vi "Compile Settings.vi"(8 "error in":errorcluster, 10 "Settings(JSON)":string, 11 "iPluginSettings in":refnum<class "Template Deployment Hooks.lvclass">) -> (0 "error out":errorcluster, 2 "Compiled Settings":variant, 3 "iPluginSettings out":refnum<class "Template Deployment Hooks.lvclass">)   [LabVIEW 2026, in "Template Deployment Hooks.lvlib" / "Template Deployment Hooks.lvclass"]
uses:
  Template Deployment Hooks.lvclass
  Template Deployment Hooks.lvclass/Template Deployment Hooks.ctl
  <vilib>/JDP Science/JSONtext/JSONtext.lvlib
  Shared/Compiled.Settings.ctl
  Shared/GroupedChannel.ctl
  Shared/GroupedChannelRefs.ctl
  Template Deployment Hooks.lvlib
  Shared/PluginSettings.ctl
  Shared/GroupSettings.ctl
  Shared/ChannelGroups.ctl
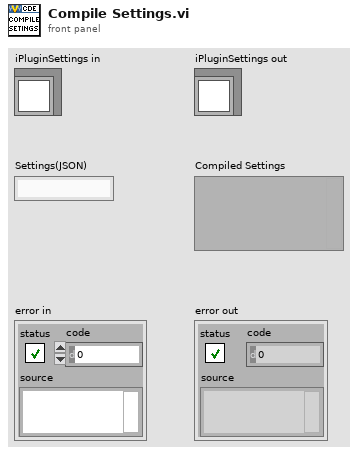
[diagram p1: front panel]
types:
  T1 = typedef "Compiled.Settings.ctl" = cluster{"Plugin Settings":T2, "Channel Groups":T3}
  T2 = typedef "PluginSettings.ctl" = cluster{"ExampleCustomDevice":cluster{"Name":string, "Properties":cluster{"Low frequency":string, "Low frequency (Hz)":bool[], "High frequency [Hz]":bool, "Frequency : Low Level frequency":dbl[], "Frequency.High frequency":dbl, "I16_PropertyExample":i16, "I16ArrayPropertyExample":i16[], "I32PropertyExample":i32, "I32ArrayPropertyExample":i32[], "I64PropertyExample":i64, "I64ArrayPropertyExample":i64[], "StringArrayPropertyExample":string[], "StringPropertyExample":string, "U16PropertyExample":u16, "U16ArrayPropertyExample":u16[], "U32PropertyExample":u32, "U32ArrayPropertyExample":u32[], "U64PropertyExample":u64, "U64ArrayPropertyExample":u64[], "DependentFilePropertyExample":cluster{"Version":string, "Type":string, "ForceDownload":bool, "RTDestination":string, "SupportedTarget":string, "MD5":string, "Path":string}, "VariantPropertyExample":variant, "TargetOS":string, "TargetRate":dbl}, "Channels":cluster{"TimeChannel":cluster{"Name":string, "Properties":cluster{"Low frequency":string, "Low frequency (Hz)":bool[], "High frequency [Hz]":bool, "Frequency : Low Level frequency":dbl[], "Frequency.High frequency":dbl, "I16PropertyExample":i16, "I16ArrayPropertyExample":i16[], "I32PropertyExample":i32, "I32ArrayPropertyExample":i32[], "I64PropertyExample":i64, "I64ArrayPropertyExample":i64[], "StringArrayPropertyExample":string[], "StringPropertyExample":string, "U16PropertyExample":u16, "U16ArrayPropertyExample":u16[], "U32PropertyExample":u32, "U32ArrayPropertyExample":u32[], "U64PropertyExample":u64, "U64ArrayPropertyExample":u64[], "DependentFilePropertyExample":cluster{"Version":string, "Type":string, "ForceDownload":bool, "RTDestination":string, "SupportedTarget":string, "MD5":string, "Path":string}, "VariantPropertyExample":variant}, "DefaultValue":dbl, "Units":string, "GroupName":string, "Type":string, "Faultable":bool, "Scalable":bool, "ChannelDataReference":i32}[], "FrequencyChannel":cluster{"Name":string, "Properties":cluster{"BinaryStringPropertyExample":string, "BooleanArrayPropertyExample":bool[], "BooleanPropertyExample":bool, "DoubleArrayPropertyExample":dbl[], "DoublePropertyExample":dbl, "I16PropertyExample":i16, "I16ArrayPropertyExample":i16[], "I32PropertyExample":i32, "I32ArrayPropertyExample":i32[], "I64PropertyExample":i64, "I64ArrayPropertyExample":i64[], "StringArrayPropertyExample":string[], "StringPropertyExample":string, "U16PropertyExample":u16, "U16ArrayPropertyExample":u16[], "U32PropertyExample":u32, "U32ArrayPropertyExample":u32[], "U64PropertyExample":u64, "U64ArrayPropertyExample":u64[], "DependentFilePropertyExample":cluster{"Version":string, "Type":string, "ForceDownload":bool, "RTDestination":string, "SupportedTarget":string, "MD5":string, "Path":string}, "VariantPropertyExample":variant}, "DefaultValue":dbl, "Units":string, "GroupName":string, "Type":string, "Faultable":bool, "Scalable":bool, "ChannelDataReference":i32}[]}, "Waveforms":cluster{"AnalogInput":cluster{"Name":string, "Properties":cluster{"Low frequency":string, "Low frequency (Hz)":bool[], "High frequency [Hz]":bool, "Frequency : Low Level frequency":dbl[], "Frequency.High frequency":dbl, "I16PropertyExample":i16, "I16ArrayPropertyExample":i16[], "I32PropertyExample":i32, "I32ArrayPropertyExample":i32[], "I64PropertyExample":i64, "I64ArrayPropertyExample":i64[], "StringArrayPropertyExample":string[], "StringPropertyExample":string, "U16PropertyExample":u16, "U16ArrayPropertyExample":u16[], "U32PropertyExample":u32, "U32ArrayPropertyExample":u32[], "U64PropertyExample":u64, "U64ArrayPropertyExample":u64[], "DependentFilePropertyExample":cluster{"Version":string, "Type":string, "ForceDownload":bool, "RTDestination":string, "SupportedTarget":string, "MD5":string, "Path":string}, "VariantPropertyExample":variant}, "DataType":string, "Units":string, "WaveformDataReference":i32}[]}, "Sections":cluster{"SectionA0":cluster{"Name":string, "Properties":cluster{"BinaryStringPropertyExample":string, "BooleanArrayPropertyExample":bool[], "BooleanPropertyExample":bool, "DoubleArrayPropertyExample":dbl[], "DoublePropertyExample":dbl, "I16PropertyExample":i16, "I16ArrayPropertyExample":i16[], "I32PropertyExample":i32, "I32ArrayPropertyExample":i32[], "I64PropertyExample":i64, "I64ArrayPropertyExample":i64[], "StringArrayPropertyExample":string[], "StringPropertyExample":string, "U16PropertyExample":u16, "U16ArrayPropertyExample":u16[], "U32PropertyExample":u32, "U32ArrayPropertyExample":u32[], "U64PropertyExample":u64, "U64ArrayPropertyExample":u64[], "DependentFilePropertyExample":cluster{"Version":string, "Type":string, "ForceDownload":bool, "RTDestination":string, "SupportedTarget":string, "MD5":string, "Path":string}, "VariantPropertyExample":variant}, "Channels":cluster{"TimeChannel":cluster{"Name":string, "Properties":cluster{"Low frequency":string, "Low frequency (Hz)":bool[], "High frequency [Hz]":bool, "Frequency : Low Level frequency":dbl[], "Frequency.High frequency":dbl, "I16PropertyExample":i16, "I16ArrayPropertyExample":i16[], "I32PropertyExample":i32, "I32ArrayPropertyExample":i32[], "I64PropertyExample":i64, "I64ArrayPropertyExample":i64[], "StringArrayPropertyExample":string[], "StringPropertyExample":string, "U16PropertyExample":u16, "U16ArrayPropertyExample":u16[], "U32PropertyExample":u32, "U32ArrayPropertyExample":u32[], "U64PropertyExample":u64, "U64ArrayPropertyExample":u64[], "DependentFilePropertyExample":cluster{"Version":string, "Type":string, "ForceDownload":bool, "RTDestination":string, "SupportedTarget":string, "MD5":string, "Path":string}, "VariantPropertyExample":variant}, "DefaultValue":dbl, "Units":string, "GroupName":string, "Type":string, "Faultable":bool, "Scalable":bool, "ChannelDataReference":i32}[], "FrequencyChannel":cluster{"Name":string, "Properties":cluster{"BinaryStringPropertyExample":string, "BooleanArrayPropertyExample":bool[], "BooleanPropertyExample":bool, "DoubleArrayPropertyExample":dbl[], "DoublePropertyExample":dbl, "I16PropertyExample":i16, "I16ArrayPropertyExample":i16[], "I32PropertyExample":i32, "I32ArrayPropertyExample":i32[], "I64PropertyExample":i64, "I64ArrayPropertyExample":i64[], "StringArrayPropertyExample":string[], "StringPropertyExample":string, "U16PropertyExample":u16, "U16ArrayPropertyExample":u16[], "U32PropertyExample":u32, "U32ArrayPropertyExample":u32[], "U64PropertyExample":u64, "U64ArrayPropertyExample":u64[], "DependentFilePropertyExample":cluster{"Version":string, "Type":string, "ForceDownload":bool, "RTDestination":string, "SupportedTarget":string, "MD5":string, "Path":string}, "VariantPropertyExample":variant}, "DefaultValue":dbl, "Units":string, "GroupName":string, "Type":string, "Faultable":bool, "Scalable":bool, "ChannelDataReference":i32}[]}, "Waveforms":cluster{"AnalogInput":cluster{"Name":string, "Properties":cluster{"Low frequency":string, "Low frequency (Hz)":bool[], "High frequency [Hz]":bool, "Frequency : Low Level frequency":dbl[], "Frequency.High frequency":dbl, "I16PropertyExample":i16, "I16ArrayPropertyExample":i16[], "I32PropertyExample":i32, "I32ArrayPropertyExample":i32[], "I64PropertyExample":i64, "I64ArrayPropertyExample":i64[], "StringArrayPropertyExample":string[], "StringPropertyExample":string, "U16PropertyExample":u16, "U16ArrayPropertyExample":u16[], "U32PropertyExample":u32, "U32ArrayPropertyExample":u32[], "U64PropertyExample":u64, "U64ArrayPropertyExample":u64[], "DependentFilePropertyExample":cluster{"Version":string, "Type":string, "ForceDownload":bool, "RTDestination":string, "SupportedTarget":string, "MD5":string, "Path":string}, "VariantPropertyExample":variant}, "DataType":string, "Units":string, "WaveformDataReference":i32}[]}}[], "SectionR1":cluster{"Name":string, "Properties":cluster{"Low frequency":string, "Low frequency (Hz)":bool[], "High frequency [Hz]":bool, "Frequency : Low Level frequency":dbl[], "Frequency.High frequency":dbl, "I16PropertyExample":i16, "I16ArrayPropertyExample":i16[], "I32PropertyExample":i32, "I32ArrayPropertyExample":i32[], "I64PropertyExample":i64, "I64ArrayPropertyExample":i64[], "StringArrayPropertyExample":string[], "StringPropertyExample":string, "U16PropertyExample":u16, "U16ArrayPropertyExample":u16[], "U32PropertyExample":u32, "U32ArrayPropertyExample":u32[], "U64PropertyExample":u64, "U64ArrayPropertyExample":u64[], "DependentFilePropertyExample":cluster{"Version":string, "Type":string, "ForceDownload":bool, "RTDestination":string, "SupportedTarget":string, "MD5":string, "Path":string}, "VariantPropertyExample":variant}, "Channels":cluster{"TimeChannel":cluster{"Name":string, "Properties":cluster{"Low frequency":string, "Low frequency (Hz)":bool[], "High frequency [Hz]":bool, "Frequency : Low Level frequency":dbl[], "Frequency.High frequency":dbl, "I16PropertyExample":i16, "I16ArrayPropertyExample":i16[], "I32PropertyExample":i32, "I32ArrayPropertyExample":i32[], "I64PropertyExample":i64, "I64ArrayPropertyExample":i64[], "StringArrayPropertyExample":string[], "StringPropertyExample":string, "U16PropertyExample":u16, "U16ArrayPropertyExample":u16[], "U32PropertyExample":u32, "U32ArrayPropertyExample":u32[], "U64PropertyExample":u64, "U64ArrayPropertyExample":u64[], "DependentFilePropertyExample":cluster{"Version":string, "Type":string, "ForceDownload":bool, "RTDestination":string, "SupportedTarget":string, "MD5":string, "Path":string}, "VariantPropertyExample":variant}, "DefaultValue":dbl, "Units":string, "GroupName":string, "Type":string, "Faultable":bool, "Scalable":bool, "ChannelDataReference":i32}[], "FrequencyChannel":cluster{"Name":string, "Properties":cluster{"BinaryStringPropertyExample":string, "BooleanArrayPropertyExample":bool[], "BooleanPropertyExample":bool, "DoubleArrayPropertyExample":dbl[], "DoublePropertyExample":dbl, "I16PropertyExample":i16, "I16ArrayPropertyExample":i16[], "I32PropertyExample":i32, "I32ArrayPropertyExample":i32[], "I64PropertyExample":i64, "I64ArrayPropertyExample":i64[], "StringArrayPropertyExample":string[], "StringPropertyExample":string, "U16PropertyExample":u16, "U16ArrayPropertyExample":u16[], "U32PropertyExample":u32, "U32ArrayPropertyExample":u32[], "U64PropertyExample":u64, "U64ArrayPropertyExample":u64[], "DependentFilePropertyExample":cluster{"Version":string, "Type":string, "ForceDownload":bool, "RTDestination":string, "SupportedTarget":string, "MD5":string, "Path":string}, "VariantPropertyExample":variant}, "DefaultValue":dbl, "Units":string, "GroupName":string, "Type":string, "Faultable":bool, "Scalable":bool, "ChannelDataReference":i32}[]}, "Sections":cluster{"SectionA0":cluster{"Name":string, "Properties":cluster{"BinaryStringPropertyExample":string, "BooleanArrayPropertyExample":bool[], "BooleanPropertyExample":bool, "DoubleArrayPropertyExample":dbl[], "DoublePropertyExample":dbl, "I16PropertyExample":i16, "I16ArrayPropertyExample":i16[], "I32PropertyExample":i32, "I32ArrayPropertyExample":i32[], "I64PropertyExample":i64, "I64ArrayPropertyExample":i64[], "StringArrayPropertyExample":string[], "StringPropertyExample":string, "U16PropertyExample":u16, "U16ArrayPropertyExample":u16[], "U32PropertyExample":u32, "U32ArrayPropertyExample":u32[], "U64PropertyExample":u64, "U64ArrayPropertyExample":u64[], "DependentFilePropertyExample":cluster{"Version":string, "Type":string, "ForceDownload":bool, "RTDestination":string, "SupportedTarget":string, "MD5":string, "Path":string}, "VariantPropertyExample":variant}, "Channels":cluster{"TimeChannel":cluster{"Name":string, "Properties":cluster{"Low frequency":string, "Low frequency (Hz)":bool[], "High frequency [Hz]":bool, "Frequency : Low Level frequency":dbl[], "Frequency.High frequency":dbl, "I16PropertyExample":i16, "I16ArrayPropertyExample":i16[], "I32PropertyExample":i32, "I32ArrayPropertyExample":i32[], "I64PropertyExample":i64, "I64ArrayPropertyExample":i64[], "StringArrayPropertyExample":string[], "StringPropertyExample":string, "U16PropertyExample":u16, "U16ArrayPropertyExample":u16[], "U32PropertyExample":u32, "U32ArrayPropertyExample":u32[], "U64PropertyExample":u64, "U64ArrayPropertyExample":u64[], "DependentFilePropertyExample":cluster{"Version":string, "Type":string, "ForceDownload":bool, "RTDestination":string, "SupportedTarget":string, "MD5":string, "Path":string}, "VariantPropertyExample":variant}, "DefaultValue":dbl, "Units":string, "GroupName":string, "Type":string, "Faultable":bool, "Scalable":bool, "ChannelDataReference":i32}[], "FrequencyChannel":cluster{"Name":string, "Properties":cluster{"BinaryStringPropertyExample":string, "BooleanArrayPropertyExample":bool[], "BooleanPropertyExample":bool, "DoubleArrayPropertyExample":dbl[], "DoublePropertyExample":dbl, "I16PropertyExample":i16, "I16ArrayPropertyExample":i16[], "I32PropertyExample":i32, "I32ArrayPropertyExample":i32[], "I64PropertyExample":i64, "I64ArrayPropertyExample":i64[], "StringArrayPropertyExample":string[], "StringPropertyExample":string, "U16PropertyExample":u16, "U16ArrayPropertyExample":u16[], "U32PropertyExample":u32, "U32ArrayPropertyExample":u32[], "U64PropertyExample":u64, "U64ArrayPropertyExample":u64[], "DependentFilePropertyExample":cluster{"Version":string, "Type":string, "ForceDownload":bool, "RTDestination":string, "SupportedTarget":string, "MD5":string, "Path":string}, "VariantPropertyExample":variant}, "DefaultValue":dbl, "Units":string, "GroupName":string, "Type":string, "Faultable":bool, "Scalable":bool, "ChannelDataReference":i32}[]}, "Waveforms":cluster{"AnalogInput":cluster{"Name":string, "Properties":cluster{"Low frequency":string, "Low frequency (Hz)":bool[], "High frequency [Hz]":bool, "Frequency : Low Level frequency":dbl[], "Frequency.High frequency":dbl, "I16PropertyExample":i16, "I16ArrayPropertyExample":i16[], "I32PropertyExample":i32, "I32ArrayPropertyExample":i32[], "I64PropertyExample":i64, "I64ArrayPropertyExample":i64[], "StringArrayPropertyExample":string[], "StringPropertyExample":string, "U16PropertyExample":u16, "U16ArrayPropertyExample":u16[], "U32PropertyExample":u32, "U32ArrayPropertyExample":u32[], "U64PropertyExample":u64, "U64ArrayPropertyExample":u64[], "DependentFilePropertyExample":cluster{"Version":string, "Type":string, "ForceDownload":bool, "RTDestination":string, "SupportedTarget":string, "MD5":string, "Path":string}, "VariantPropertyExample":variant}, "DataType":string, "Units":string, "WaveformDataReference":i32}[]}}[]}}[]}}}
  T3 = typedef "ChannelGroups.ctl" = cluster{"Channel Refs":T4, "Group Settings":T5[]}
  T4 = typedef "GroupedChannelRefs.ctl" = cluster{"Read":cluster{"Refs":cluster{"Data Reference":i32, "Offset":u64, "Length":u64}[], "Values":dbl[]}[], "Write":cluster{"Refs":cluster{"Data Reference":i32, "Offset":u64, "Length":u64}[], "Values":dbl[]}[], "ReadWrite":cluster{"Refs":i32[], "Values":dbl[], "Reset Values":dbl[]}[], "LUT":variant}
  T5 = typedef "GroupSettings.ctl" = cluster{"Name":string, "Channel Type":enum16{"Output/Write", "Input/Read", "Input/ReadWrite"}, "Channel Settings":T6[]}
  T6 = typedef "GroupedChannel.ctl" = cluster{"Name":string, "TypeName":string, "ChannelProperties":variant}
  T7 = cluster{"Channel Refs":cluster{"Read":cluster{"Refs":cluster{"Data Reference":i32, "Offset":u64, "Length":u64}[], "Values":dbl[]}[], "Write":cluster{"Refs":cluster{"Data Reference":i32, "Offset":u64, "Length":u64}[], "Values":dbl[]}[], "ReadWrite":cluster{"Refs":i32[], "Values":dbl[], "Reset Values":dbl[]}[], "LUT":variant}, "GroupSettings":cluster{"Name":string, "ChannelSettings":cluster{"Name":string, "TypeName":string, "ChannelProperties":variant}[]}[]}
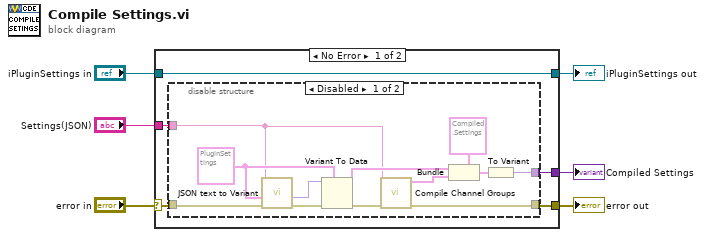
[diagram p0: block diagram]
diagram:
  n1 = case shown="No Error" "error in" {
    selector: "error in" -> [w11 w26]
    tunnel: "Settings(JSON)" -> [w8 _]
    tunnel: [w9 _] -> w3
    tunnel: [w10 w26] -> w5
    tunnel: [w7 w25] -> w2
    tunnel: "iPluginSettings in" -> [w7 w25]
    frame No Error {
      n2 = disable-structure shown="Disabled" {
        disable-tunnel: w11 -> [w23 w24]
        disable-tunnel: [w18 _] -> w9
        disable-tunnel: w8 -> [w13 _]
        disable-tunnel: [w20 w24] -> w10
        frame Disabled {
          w17 = T2 {"ExampleCustomDevice"={"Name"="", "Properties"={"Low frequency"="", "Low frequency (Hz)"=[], "High frequency [Hz]"=FALSE, "Frequency : Low Level frequency"=[], "Frequency.High frequency"=0.0, "I16_PropertyExample"=0, "I16ArrayPropertyExample"=[], "I32PropertyExample"=0, "I32ArrayPropertyExample"=[], "I64PropertyExample"=0, "I64ArrayPropertyExample"=[], "StringArrayPropertyExample"=[], "StringPropertyExample"="", "U16PropertyExample"=0, "U16ArrayPropertyExample"=[], "U32PropertyExample"=0, "U32ArrayPropertyExample"=[], "U64PropertyExample"=0, "U64ArrayPropertyExample"=[], "DependentFilePropertyExample"={"Version"="", "Type"="", "ForceDownload"=FALSE, "RTDestination"="", "SupportedTarget"="", "MD5"="", "Path"=""}, "VariantPropertyExample"=variant, "TargetOS"="", "TargetRate"=0.0}, "Channels"={"TimeChannel"=[], "FrequencyChannel"=[]}, "Waveforms"={"AnalogInput"=[]}, "Sections"={"SectionA0"=[], "SectionR1"=[]}}} ("PluginSettings")
          n3 = call <vilib>:"JSON text to Variant.vi"("error in (no error)"=w23, "Data Type"=w17, "JSON"=w13) -> ("error out"=w22:errorcluster, "Variant out"=w19:variant)  [unwired: 7 in]
          n4 = Variant To Data(error in=w22, type=w17, Variant=w19) -> (data=w15:T2, error out=w21:errorcluster)
          n5 = call "Compile Channel Groups.vi"("error in"=w21, "Settings(JSON)"=w13) -> ("error out"=w20:errorcluster, "ChannelGroups"=w12:T7)  [unwired: 8 in]
          n6 = Bundle(cluster=T1 {"Plugin Settings"={"ExampleCustomDevice"={"Name"="", "Properties"={"Low frequency"="", "Low frequency (Hz)"=[], "High frequency [Hz]"=FALSE, "Frequency : Low Level frequency"=[], "Frequency.High frequency"=0.0, "I16_PropertyExample"=0, "I16ArrayPropertyExample"=[], "I32PropertyExample"=0, "I32ArrayPropertyExample"=[], "I64PropertyExample"=0, "I64ArrayPropertyExample"=[], "StringArrayPropertyExample"=[], "StringPropertyExample"="", "U16PropertyExample"=0, "U16ArrayPropertyExample"=[], "U32PropertyExample"=0, "U32ArrayPropertyExample"=[], "U64PropertyExample"=0, "U64ArrayPropertyExample"=[], "DependentFilePropertyExample"={"Version"="", "Type"="", "ForceDownload"=FALSE, "RTDestination"="", "SupportedTarget"="", "MD5"="", "Path"=""}, "VariantPropertyExample"=variant, "TargetOS"="", "TargetRate"=0.0}, "Channels"={"TimeChannel"=[], "FrequencyChannel"=[]}, "Waveforms"={"AnalogInput"=[]}, "Sections"={"SectionA0"=[], "SectionR1"=[]}}}, "Channel Groups"={"Channel Refs"={"Read"=[], "Write"=[], "ReadWrite"=[], "LUT"=variant}, "Group Settings"=[]}} ("CompiledSettings"), "Plugin Settings"=w15, "Channel Groups"=w12) -> (w14:T1)
          n7 = To Variant(anything=w14) -> (Variant=w18:variant)
        }
        frame Enabled {
        }
      }
    }
    frame Error {
    }
  }
  "error out" <- w5
  "iPluginSettings out" <- w2
  "Compiled Settings" <- w3
